vi "生成索引.vi"(11 "data out输入":string) -> (1 "OK":bool, 2 "行":i32, 3 "列":i32)   [LabVIEW 2011]
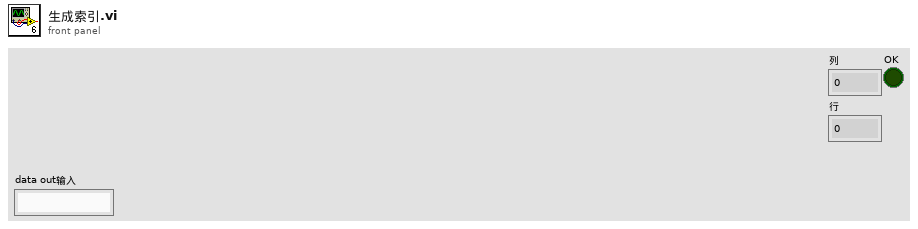
[diagram p1: front panel]
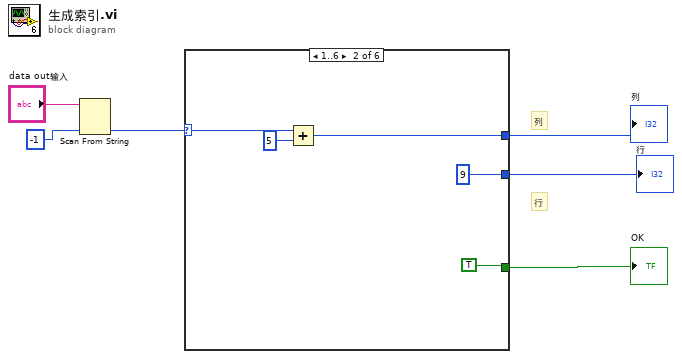
[diagram p0: block diagram]
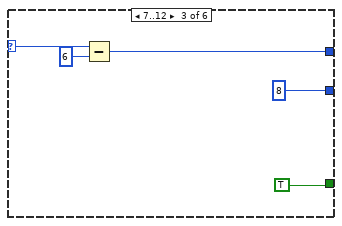
[diagram p3: hidden frame]
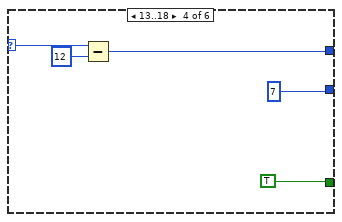
[diagram p4: hidden frame]
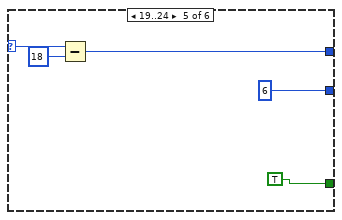
[diagram p5: hidden frame]
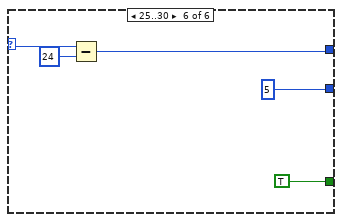
[diagram p6: hidden frame]
diagram:
  # "行"
  # "列"
  n1 = Scan From String(input string="data out输入", default 1=-1) -> (output 1=w4:i32)  [unwired: 3 in, 3 out]
  n2 = case shown="1..6" w4 {
    selector: w4 -> [_ w11 w16 w21 w26 w31]
    tunnel: [_ w9 w14 w20 w24 w30] -> w3
    tunnel: [_ 9 8 7 ("y") 6 5] -> w2
    tunnel: [_ TRUE TRUE TRUE TRUE TRUE] -> w1
    frame 0, Default {
    }
    frame 1..6 {
      n3 = Add(x=w11, y=5) -> (x+y=w9:i32)
    }
    frame 7..12 {
      n4 = Subtract(x=w16, y=6) -> (x-y=w14:i32)
    }
    frame 13..18 {
      n5 = Subtract(x=w21, y=12) -> (x-y=w20:i32)
    }
    frame 19..24 {
      n6 = Subtract(x=w26, y=18) -> (x-y=w24:i32)
    }
    frame 25..30 {
      n7 = Subtract(x=w31, y=24) -> (x-y=w30:i32)
    }
  }
  "列" <- w3
  "行" <- w2
  "OK" <- w1
